vi "_recreate obj.vi"(9 "Array":string[][](array[string]), 10 "columns data type":string[](array[string]), 11 "_ISerializable in":refnum<class "_ISerializable.lvclass">) -> (2 "Array 3":T1[][](array[typedef]), 3 "data":string[][](array[string]))   [LabVIEW 2018, in "LV-ORM.lvclass"]
uses:
  LV-ORM.lvclass
  _Serializable Base Object/_ISerializable.lvclass
  Typedefs/key-value-type cluster.ctl
  Serializer/Serializer.lvclass
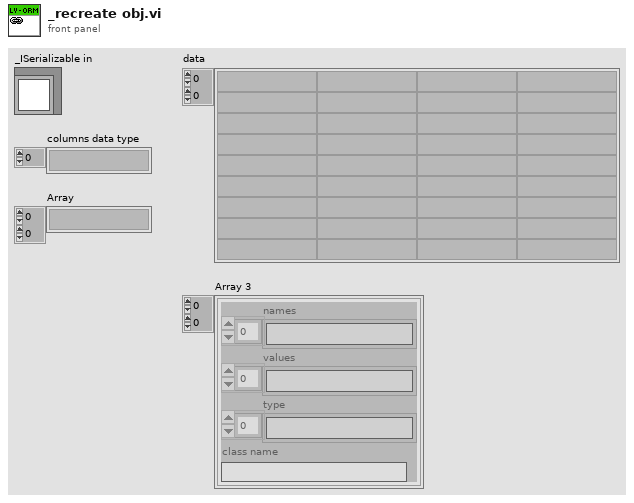
[diagram p1: front panel]
types:
  T1 = typedef "key-value-type cluster.ctl" = cluster{"names":string[], "values":string[], "type":string[], "class name":string}
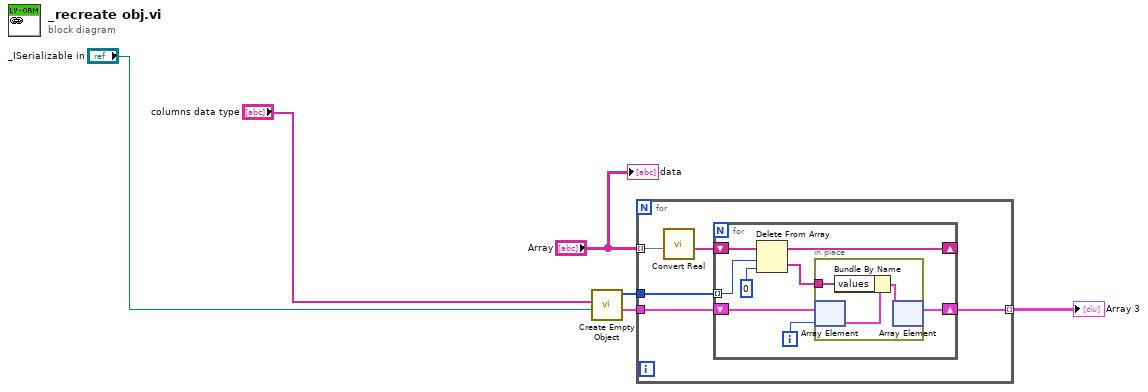
[diagram p0: block diagram]
diagram:
  n1 = call "Create Empty Object.vi"("object"="_ISerializable in", "columns data type"="columns data type") -> ("Array 3"=w4:T1[], "elements by level"=w3:i32[])  [unwired: 8 in]
  n2 = for {
    tunnel: "Array" -> [w8] mode=indexing
    tunnel: [w11] -> w2 mode=indexing
    tunnel: w3 -> [w10]
    tunnel: w4 -> [w9]
    n3 = call "Convert Real.vi"("data in"=w8) -> ("data out"=w7:string[])  [unwired: 10 in]
    n4 = for {
      shift-right: [w12] -> w11
      shift-left: w9 -> [w17]
      shift-right: [w14] -> _
      shift-left: w7 -> [w19]
      tunnel: w10 -> [w18] mode=indexing
      i -> [w16]
      n5 = Delete From Array(array=w19, length=w18, index=0) -> (deleted portion=w15:string[], array with subset deleted=w14:string[])
      n6 = in-place {
        in-place-border: w15 -> [w20]
        n7 = in-place-array #1(w17, w16) -> (w22:T1)
        n8 = Bundle By Name(cluster=w22, "values"=w20) -> (w21:T1)
        n9 = in-place-array #1(w21) -> (w12:T1[])  [unwired: 1 out]
      }
    }
  }
  "Array 3" <- w2
  "data" <- "Array"
